vi "컴퓨터이름.vi"() -> ()   [LabVIEW 2014]
uses:
  kernel32.dll
panel:
  out "ComputerName":string
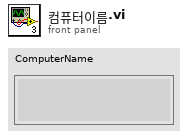
[diagram p1: front panel]
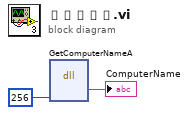
[diagram p0: block diagram]
diagram:
  n1 = dll-call lib="kernel32.dll" fn="GetComputerNameA"("len"=u32 256) -> ("ComputerName"=→"ComputerName":string)  [unwired: 6 in, 2 out]
